vi "Set Source Power Start.vi"(7 "Start":dbl, 8 "error in (no error)":errorcluster {"code" format="%.0x"}, 9 "PortVal":i32 format="%.0g", 10 "Channel":string, 11 "instrument handle":refnum<k15>) -> (0 "error out":errorcluster {"code" format="%.0x"}, 3 "instrument handle out":refnum<k15>)   [LabVIEW 2014, in "Agilent NA.lvlib"]
doc: "Sets/Get the power sweep start power"
uses:
  Agilent NA.lvlib
  AgNA.dll
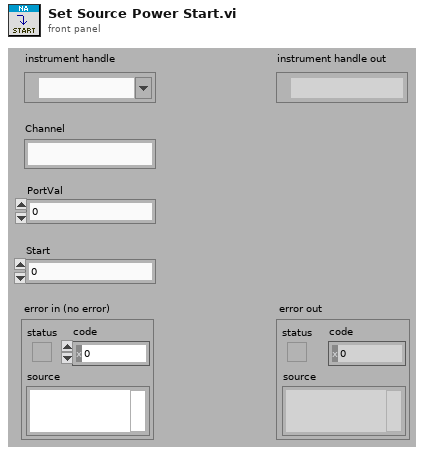
[diagram p1: front panel]
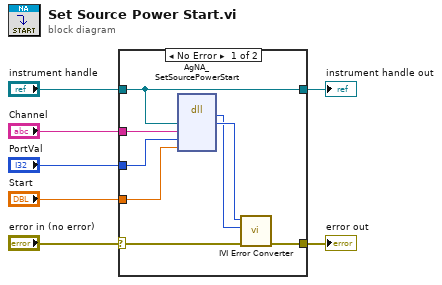
[diagram p0: block diagram]
diagram:
  n1 = case shown="No Error" "error in (no error)" {
    selector: "error in (no error)" -> [w13 w17]
    tunnel: [w12 w17] -> w7
    tunnel: "Channel" -> [w11 _]
    tunnel: "PortVal" -> [w10 _]
    tunnel: "Start" -> [w9 _]
    tunnel: [w8 w16] -> w2
    tunnel: "instrument handle" -> [w8 w16]
    frame No Error {
      n2 = dll-call lib="AgNA**.dll" fn="AgNA_SetSourcePowerStart"("Vi"=w8, "Channel"=w11, "PortVal"=w10, "Start"=w9) -> (w14:i32, "Vi"=w15:u32)  [unwired: 6 in, 2 out]
      n3 = call "IVI Error Converter.vi"("error in (no error)"=w13, "IVI error code (0)"=w14, "instrument handle"=w15) -> ("error out"=w12:errorcluster)  [unwired: 7 in, 1 out]
    }
    frame Error {
    }
  }
  "error out" <- w7
  "instrument handle out" <- w2
